vi "Read Actual Sample Information.vi"(8 "error in (no error)":errorcluster, 11 "VISA resource name":refnum<visa-resource-name>) -> (0 "error out":errorcluster, 1 "Sample Mode":string, 2 "Sample Rate":dbl, 3 "VISA resource name out":refnum<visa-resource-name>)   [LabVIEW 2017, in "Agilent 6000 Series.lvlib"]
doc: "This VI returns the effective sample rate of the acquired waveform using the current configuration in samples per second and the sample mode the oscilloscope is currently using."
uses:
  <instrlib>/Agilent 6000 Series/Agilent 6000 Series.lvlib
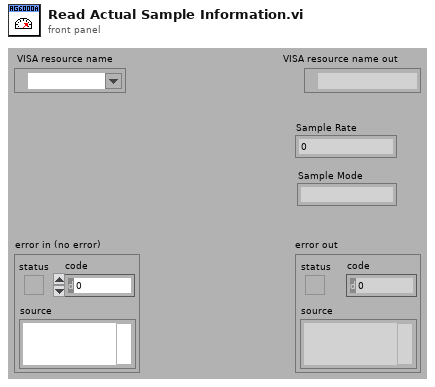
[diagram p1: front panel]
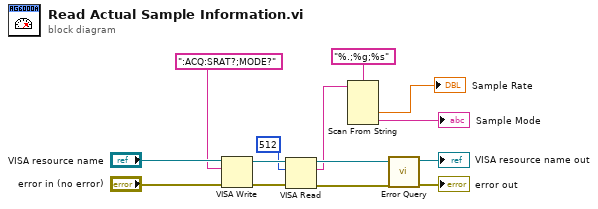
[diagram p0: block diagram]
diagram:
  n1 = VISA Write(VISA resource name="VISA resource name", write buffer=":ACQ:SRAT?;MODE?", error in (no error)="error in (no error)") -> (VISA resource name out=w6:refnum<visa-resource-name>, error out=w9:errorcluster)  [unwired: 1 out]
  n2 = VISA Read(VISA resource name=w6, byte count=u32 512, error in (no error)=w9) -> (VISA resource name out=w7:refnum<visa-resource-name>, read buffer=w4:string, error out=w8:errorcluster)  [unwired: 1 out]
  n3 = Scan From String(format string="%.;%g;%s", input string=w4) -> (output 1=→"Sample Rate":dbl, output 2=→"Sample Mode":string)  [unwired: 4 in, 3 out]
  n4 = call <instrlib>:"Error Query.vi"("error in (no error)"=w8, "VISA resource name"=w7) -> ("error out"=→"error out":errorcluster, "VISA resource name out"=→"VISA resource name out":refnum<visa-resource-name>)  [unwired: 6 in, 2 out]
